vi "myRIO_BRig_RT_arrTrig_Cue1_CueType_AudioLed.vi"() -> (2 "output_arrTrig_Cue1_CueType_AudioLed":i32)   [LabVIEW 2014]
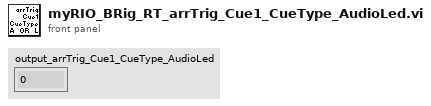
[diagram p1: front panel]
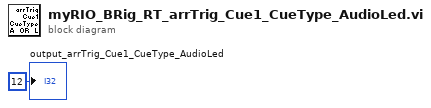
[diagram p0: block diagram]
diagram:
  "output_arrTrig_Cue1_CueType_AudioLed" <- 12
